vi "Get New Level.vi"(8 "error in (no error)":errorcluster, 11 "Cooler in":refnum<class "Cooler.lvclass">) -> (0 "error out":errorcluster, 2 "Level":dbl, 3 "Cooler out":refnum<class "Cooler.lvclass">)   [LabVIEW 2012, in "Cooler.lvlib" / "Cooler.lvclass"]
uses:
  Cooler.lvclass
  Simulation/Simulation Data_Global.vi
  Simulation/Simulation.lvlib
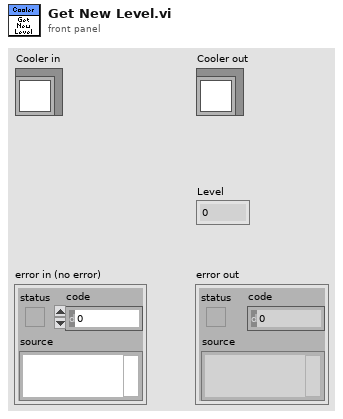
[diagram p1: front panel]
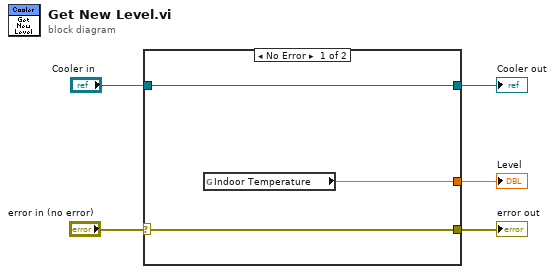
[diagram p0: block diagram]
diagram:
  n1 = case shown="No Error" "error in (no error)" {
    selector: "error in (no error)" -> [w6 _]
    tunnel: "Cooler in" -> [w7 w9]
    tunnel: [w8 _] -> w4
    tunnel: [w7 w9] -> w3
    tunnel: [w6 _] -> w1
    frame No Error {
      n2 = global read "Simulation Data_Global.vi" "Indoor Temperature"() -> (w8:dbl)
    }
    frame Error {
    }
  }
  "error out" <- w1
  "Cooler out" <- w3
  "Level" <- w4
